vi "Data headlines.vi"() -> (0 "Headlines (vertical array)":string[](array[string]))   [LabVIEW 2022 SP3]
doc: "Headlines for data generated by the computer vision"
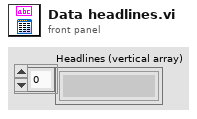
[diagram p1: front panel]
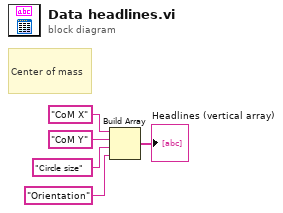
[diagram p0: block diagram]
diagram:
  # "Center of mass"
  n1 = Build Array("CoM X", "CoM Y", "Circle size" ("element"), "Orientation") -> (→"Headlines (vertical array)":string[])
